vi "Toggle on Press and Release.vi"(11 "Boolean in":bool) -> (3 "Boolean out":bool)   [LabVIEW 2018]
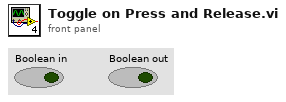
[diagram p1: front panel]
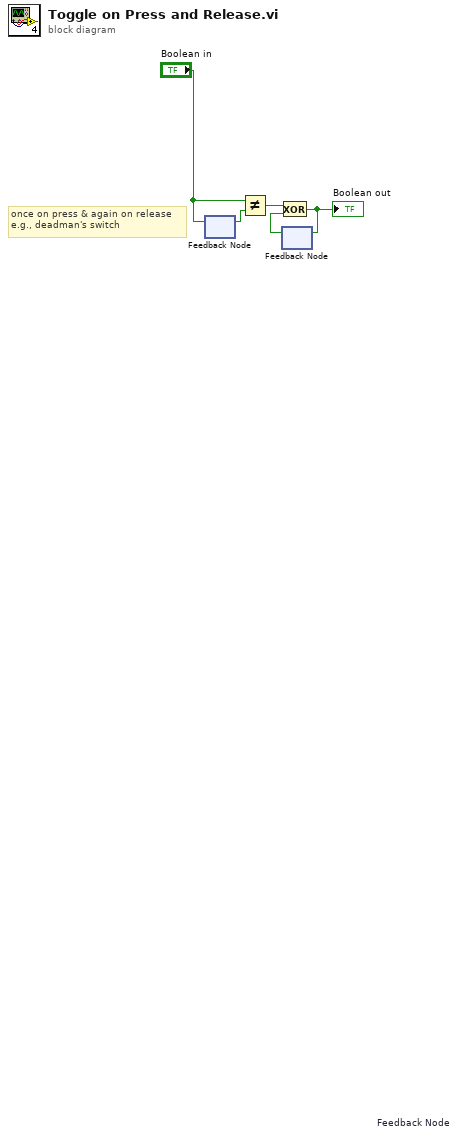
[diagram p0: block diagram]
diagram:
  # "once on press & again on release\ne.g., deadman's switch"
  n1 = feedback #1 "Feedback Node"() -> (w1:bool)  [unwired: 1 in]
  n2 = feedback-in #1("Boolean in") -> ()
  n3 = Not Equal?(x="Boolean in", y=w1) -> (x != y?=w3:bool)
  n4 = feedback #2() -> (w4:bool)  [unwired: 1 in]
  n5 = Exclusive Or(1:w4, 2:w3) -> (0:w2:bool)
  "Boolean out" <- w2
  n6 = feedback-in #2(w2) -> ()
